vi "FIle_Folder Create If Needed.vi"(8 "Error":errorcluster, 9 "Folder Name":string, 11 "Parrent Folder path":path) -> (0 "Error Out":errorcluster, 2 "Success Out":bool, 3 "Dup Path Out":path)   [LabVIEW 2020]
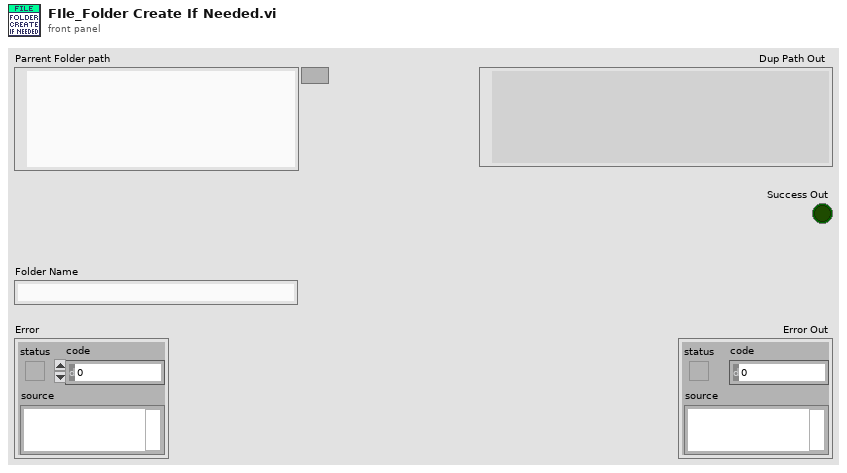
[diagram p1: front panel]
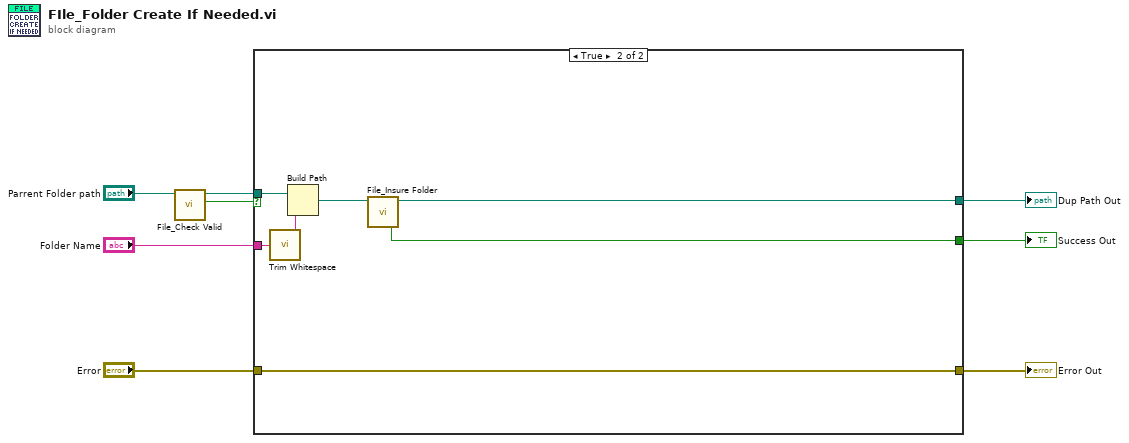
[diagram p0: block diagram]
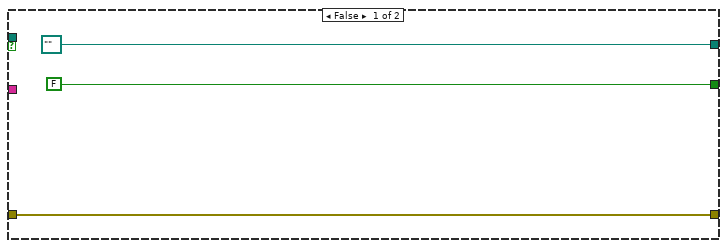
[diagram p2: hidden frame]
diagram:
  n1 = call "File_Check Valid.vi"("path"="Parrent Folder path") -> ("dup path"=w1:path, "valid"=w3:bool)  [unwired: 4 in, 1 out]
  n2 = case shown="True" w3 {
    tunnel: [w9 w14] -> w8
    tunnel: [path "" ("dup path") w12] -> w7
    tunnel: [FALSE ("file or folder exists?") w13] -> w6
    tunnel: "Error" -> [w9 w14]
    tunnel: "Folder Name" -> [_ w17]
    tunnel: w1 -> [_ w16]
    frame False {
    }
    frame True {
      n3 = call <vilib>:"Trim Whitespace.vi"("string"=w17) -> ("trimmed string"=w18:string)  [unwired: 1 in]
      n4 = Build Path(base path=w16, name or relative path=w18) -> (appended path=w15:path)
      n5 = call "File_Insure Folder.vi"("Folder"=w15) -> ("created path"=w12:path, "Success"=w13:bool)  [unwired: 3 in]
    }
  }
  "Error Out" <- w8
  "Dup Path Out" <- w7
  "Success Out" <- w6
